vi "UpdateStatus.vi"(4 "Active MFC address":i32=7, 6 "Inert MFC address":i32=8, 7 "Probe Current State":T1 {"Tset" format="%.1f"; "Telem" format="%.1f"; "GasC" format="%.1g"; "GasB" format="%.1f"; "GasA" format="%.1f"; "Z" format="%.3g"; "Y" format="%.3g"; "X" format="%.3g"; "RampRate" format="%.1f"}, 8 "error in":errorcluster, 9 "MFC Channel":refnum<visa-resource-name>="COM5", 10 "Watlow channel":refnum<visa-resource-name>="COM3", 11 "Motor channel":refnum<visa-resource-name>="COM6") -> (0 "error out":errorcluster, 1 "Chiller flow?":bool, 3 "Updated probe state":T1 {"Tset" format="%.1f"; "Telem" format="%.1f"; "GasC" format="%.1g"; "GasB" format="%.1f"; "GasA" format="%.1f"; "Z" format="%.3g"; "Y" format="%.3g"; "X" format="%.3g"; "RampRate" format="%.1f"})   [LabVIEW 2013]
uses:
  controls/Microprobe Vars.ctl
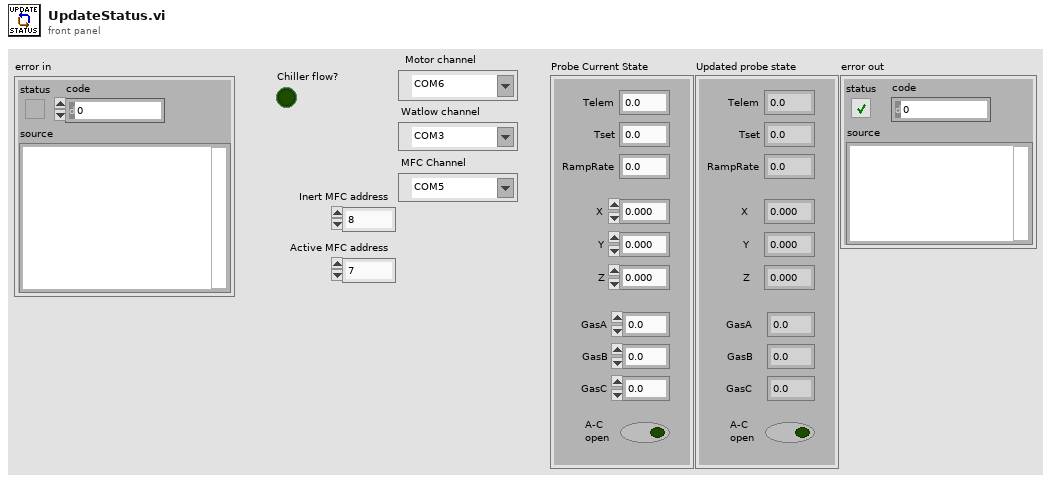
[diagram p1: front panel]
types:
  T1 = typedef "Microprobe Vars.ctl" = cluster{"Telem":dbl, "Tset":dbl, "RampRate":dbl, "X":dbl, "Y":dbl, "Z":dbl, "GasA":dbl, "GasB":dbl, "GasC":dbl, "A-C\nopen":bool}
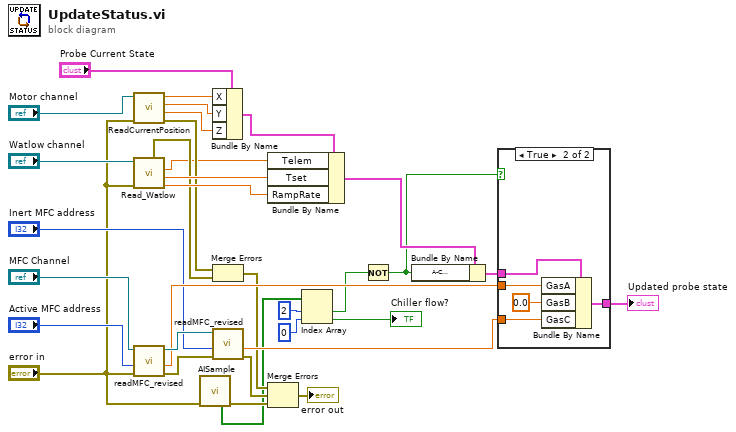
[diagram p0: block diagram]
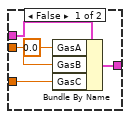
[diagram p2: hidden frame]
diagram:
  n1 = call <instrlib>:"ReadCurrentPosition.vi"("error in"="error in", "Motor channel"="Motor channel") -> ("error out"=w5:errorcluster, "Z"=w32:dbl, "Y"=w24:dbl, "X"=w25:dbl)  [unwired: 5 in, 1 out]
  n2 = call <instrlib>:"Read_Watlow.vi"("Error In"="error in", "Watlow channel"="Watlow channel") -> ("Ramp rate"=w30:dbl, "Setpoint"=w31:dbl, "Current temp"=w4:dbl, "Error Out"=w23:errorcluster)  [unwired: 4 in, 1 out]
  n3 = call <instrlib>:"readMFC_revised.vi"("error in"="error in", "channel"="Active MFC address", "VISA resource name"="MFC Channel") -> ("error out"=w33:errorcluster, "flow rate sccm"=w27:dbl, "VISA resource name out"=w28:refnum<visa-resource-name>)  [unwired: 6 in]
  n4 = call <vilib>:"AISample.vi"("error in"="error in") -> ("IO State Read"=w7:bool[], "error out"=w16:errorcluster)  [unwired: 11 in, 2 out]
  n5 = Bundle By Name(cluster="Probe Current State", "X"=w25, "Y"=w24, "Z"=w32) -> (w29:T1)
  n6 = Merge Errors(w5, w23) -> (w22:errorcluster)
  n7 = call <instrlib>:"readMFC_revised.vi"("error in"=w33, "channel"="Inert MFC address", "VISA resource name"=w28) -> ("error out"=w21:errorcluster, "flow rate sccm"=w26:dbl)  [unwired: 6 in, 1 out]
  n8 = Bundle By Name(cluster=w29, "Telem"=w4, "Tset"=w31, "RampRate"=w30) -> (w18:T1)
  n9 = Merge Errors(w22, w21, w16) -> (→"error out":errorcluster)
  n10 = Index Array(array=w7, index #1=2 ("index"), index #2=0 ("index")) -> (element #1=w1:bool, element #2=→"Chiller flow?":bool)
  n11 = Not(x=w1) -> (.not. x?=w17:bool)
  n12 = Bundle By Name(cluster=w18, "A-C\nopen"=w17) -> (w19:T1)
  n13 = case shown="True" w17 {
    tunnel: w27 -> [w38 w41]
    tunnel: w19 -> [w35 w43]
    tunnel: [w36 w42] -> w10
    tunnel: w26 -> [w34 w39]
    frame False {
      n14 = Bundle By Name(cluster=w35, "GasA"=0.0, "GasB"=w38, "GasC"=w34) -> (w36:T1)
    }
    frame True {
      n15 = Bundle By Name(cluster=w43, "GasA"=w41, "GasB"=0.0, "GasC"=w39) -> (w42:T1)
    }
  }
  "Updated probe state" <- w10
